vi "tb_SPI Engine (Host).vi"() -> ()   [LabVIEW 2014]
uses:
  user.lib/_NI SPI IP/FPGA/Controllers/Public/Spi Master Inputs.ctl
  user.lib/_NI SPI IP/FPGA/Controllers/Public/Spi Master Outputs.ctl
  user.lib/_NI SPI IP/FPGA/Controllers/Public/Transfer Settings.ctl
  user.lib/_NI SPI IP/FPGA/Controllers/NI SPI IP (FPGA).lvlib
panel:
  out "ready for input":bool
  out "SPI Signals":digitalwaveform(graph)
  in  "Loop Time(ms)":u32=5
  out "Iterations":i32
  in  "start strobe":bool
  in  "stop":bool
  in  "spi transfer settings":T1={"Divide Value"=10, "Transfer Length (bits)"=32, "CS Asserted Polarity"=FALSE, "Clock Polarity (CPOL)"=FALSE, "Clock Phase (CPHA)"=FALSE, "Lengthen MISO Setup"=FALSE, "Direction Change Bit"=0, "MOSI Starts as Output"=FALSE, "Tristatable MOSI"=FALSE} {"Direction Change Bit" max=64 step=1; "Transfer Length (bits)" min=1 max=64 step=1}
  in  "data to write":u64 format="%.0x"
  out "spi output":T2
  in  "spi input":T3
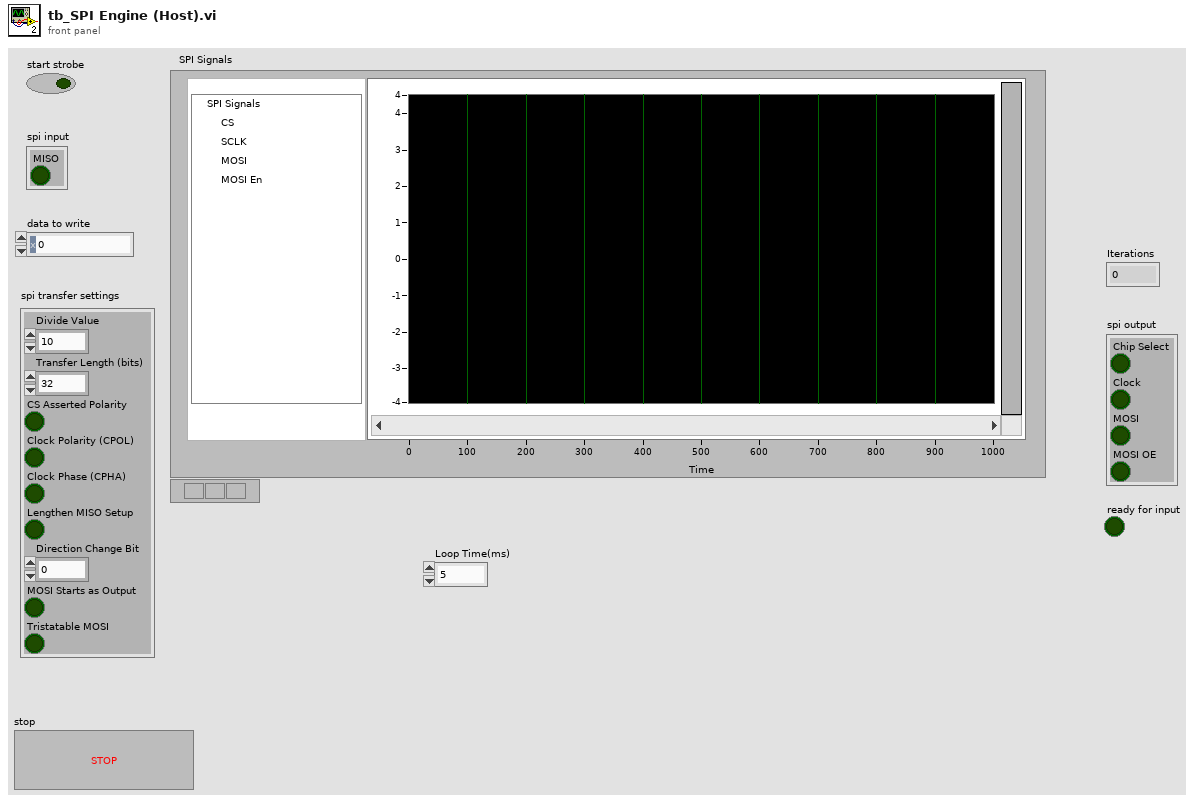
[diagram p1: front panel]
types:
  T1 = typedef "NI SPI IP (FPGA).lvlib/Transfer Settings.ctl" = cluster{"Divide Value":u8, "Transfer Length (bits)":u8, "CS Asserted Polarity":bool, "Clock Polarity (CPOL)":bool, "Clock Phase (CPHA)":bool, "Lengthen MISO Setup":bool, "Direction Change Bit":u8, "MOSI Starts as Output":bool, "Tristatable MOSI":bool}
  T2 = typedef "NI SPI IP (FPGA).lvlib/Spi Master Outputs.ctl" = cluster{"Chip Select":bool, "Clock":bool, "MOSI":bool, "MOSI OE":bool}
  T3 = typedef "NI SPI IP (FPGA).lvlib/Spi Master Inputs.ctl" = cluster{"MISO":bool}
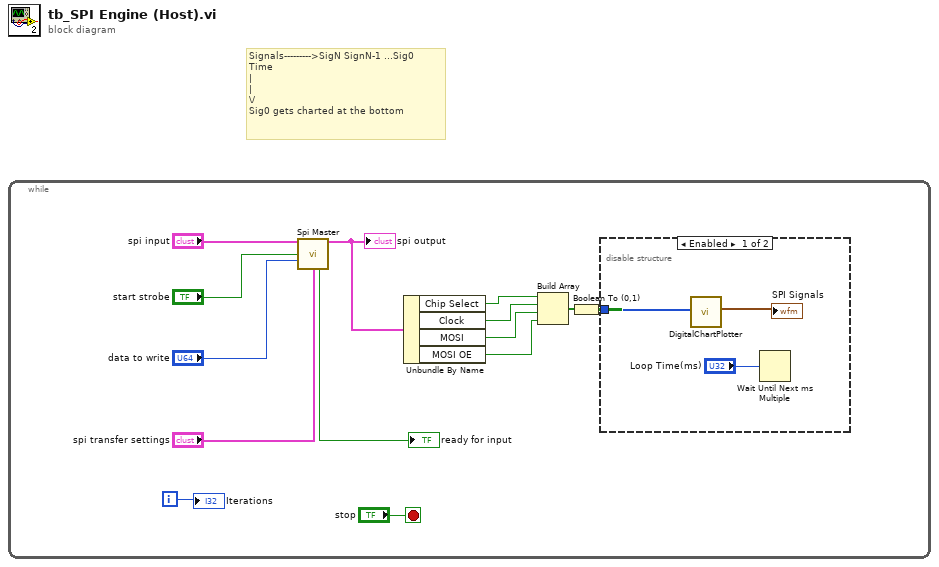
[diagram p0: block diagram]
diagram:
  # "Signals--------->SigN SignN-1 ...Sig0\nTime\n|\n|\n\\/\nSig0 gets charted at the bottom"
  n1 = while {
    i -> [w5]
    stop <- "stop" stop-if-true
    n2 = call "Spi Master.vi"("spi input"="spi input", "start strobe"="start strobe", "data to write"="data to write", "spi transfer settings"="spi transfer settings") -> ("spi output"=w9:T2, "ready for input"=→"ready for input":bool)  [unwired: 8 in, 2 out]
    "spi output" <- w9
    n3 = Unbundle By Name(w9) -> ("Chip Select"=w8:bool, "Clock"=w1:bool, "MOSI"=w7:bool, "MOSI OE"=w6:bool)
    n4 = Build Array(w8, w1, w7, w6) -> (w4:bool[])
    n5 = Boolean To (0,1)(Boolean=w4) -> (0, 1=w3:i16[])
    n6 = disable-structure shown="Enabled" {
      disable-tunnel: w3 -> [w16 _]
      frame Enabled {
        n7 = call "DigitalChartPlotter.vi"("Input"=w16) -> ("Digital Data"=→"SPI Signals":digitalwaveform)  [unwired: 10 in]
        n8 = Wait Until Next ms Multiple(millisecond multiple="Loop Time(ms)") -> ()  [unwired: 1 out]
      }
      frame Disabled {
      }
    }
    "Iterations" <- w5
  }
